vi "WPI_SolenoidSafetyCheck.vi"(0 "SolenoidDevRef":T1={"DevStatus"={"status"=FALSE, "code"=0, "source"=""}, "Pneumatics Control Module"=1, "Forward Solenoid Channel"=enum."Solenoid 1", "Reverse Solenoid Channel"=enum."Invalid"}, 5 "menu":T3, 7 "VI Refnum":refnum<vi>, 9 "timeout (ms)":u32=100, 11 "error in (no error)":errorcluster) -> (15 "error out":errorcluster)   [LabVIEW 2017]
doc: "This subVI holds an array of DevRefs, timeout values, and latest update times. These values can be added, updated, tested, and removed.\n\nThis gets called by Open to add a set of values. It gets called by Drive to update the 'last update value'. It gets called by Close to remove a set of values.\n\nIt also gets called by Safety Test via the SafetyCheckEngine that runs as a background task called by the Start Communication loop to test all sets of values for a timeout condition.\n\nThis software is licensed. Open the labview\\readme\\WPI Robotics Library Open Source License.txt file for more information."
uses:
  <vilib>/Rock Robotics/WPI/SafetyOutput/WPI_SafetyOutputCheckMenu.ctl
  <vilib>/Rock Robotics/WPI/Solenoid/WPI_SolenoidDevRef.ctl
  <vilib>/Rock Robotics/WPI/Solenoid/WPI_SolenoidChannel.ctl
  <vilib>/Rock Robotics/WPI/CAN/PCM/WPI_CAN_PCMGlobalOps.ctl
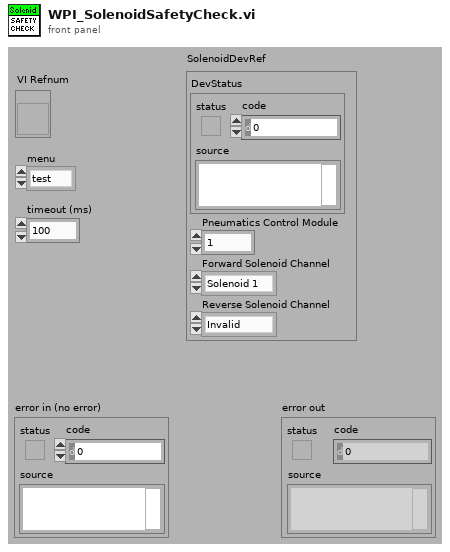
[diagram p1: front panel]
types:
  T1 = typedef "WPI_SolenoidDevRef.ctl" = cluster{"DevStatus":errorcluster, "Pneumatics Control Module":u8, "Forward Solenoid Channel":T2, "Reverse Solenoid Channel":T2}
  T2 = typedef "WPI_SolenoidChannel.ctl" = enum8{"Solenoid 0", "Solenoid 1", "Solenoid 2", "Solenoid 3", "Solenoid 4", "Solenoid 5", "Solenoid 6", "Solenoid 7", "Invalid"}
  T3 = typedef "WPI_SafetyOutputCheckMenu.ctl" = enum16{"test", "add", "remove", "update"}
  T4 = typedef "WPI_CAN_PCMGlobalOps.ctl" = enum16{"Read For Send", "Write After Receive", "Set Solenoids", "Set Closed Loop", "Clear Sticky Faults", "Get All", "Write Error", "Write After Receive Blacklist", "Set Control Frame Rate"}
  T5 = cluster{"Solenoid Status":bool[], "Battery Voltage":dbl, "Solenoid Voltage":dbl, "Compressor Current":dbl, "CompressorEnabled":bool, "StickySolenoidFault":bool, "StickyCompressorFault":bool, "SolenoidFault":bool, "CompressorFault":bool, "HardwareFault":bool, "ClosedLoopStatus":bool, "PressureStatus":bool, "Module Enabled":bool, "ClosedLoopSuggestedOutput":bool, "CAN Error":errorcluster, "Sticky Solenoid Faults":bool[]}
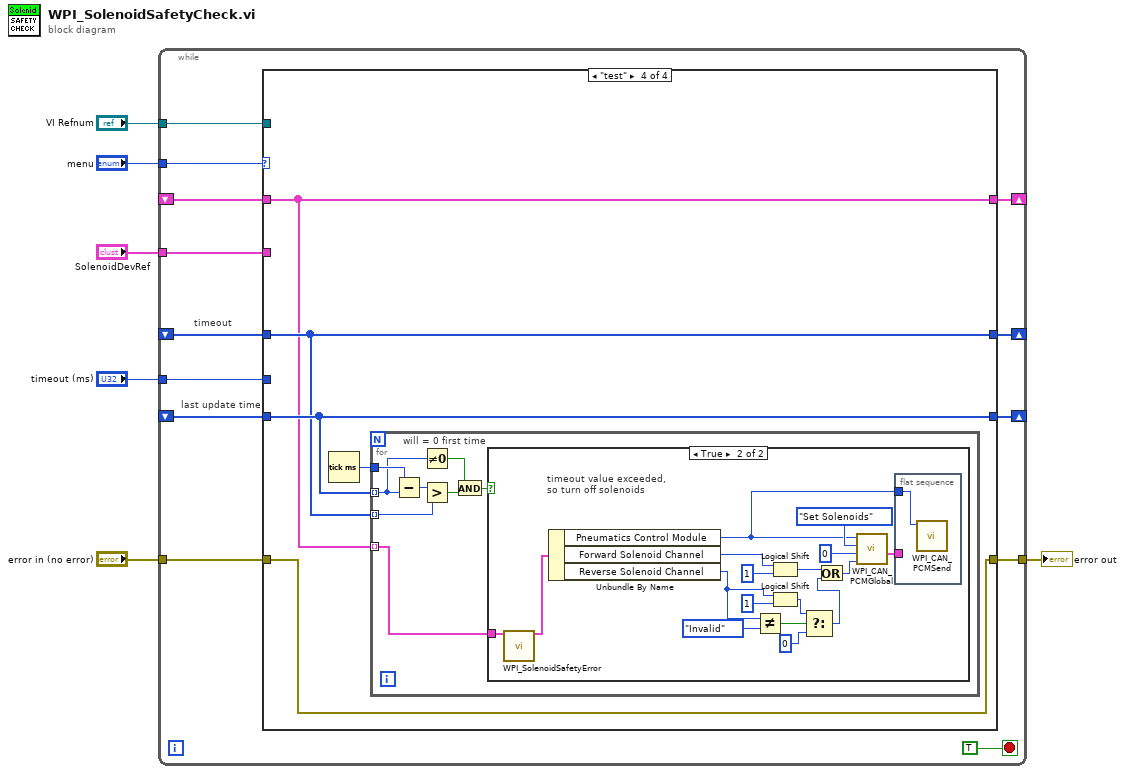
[diagram p0: block diagram]
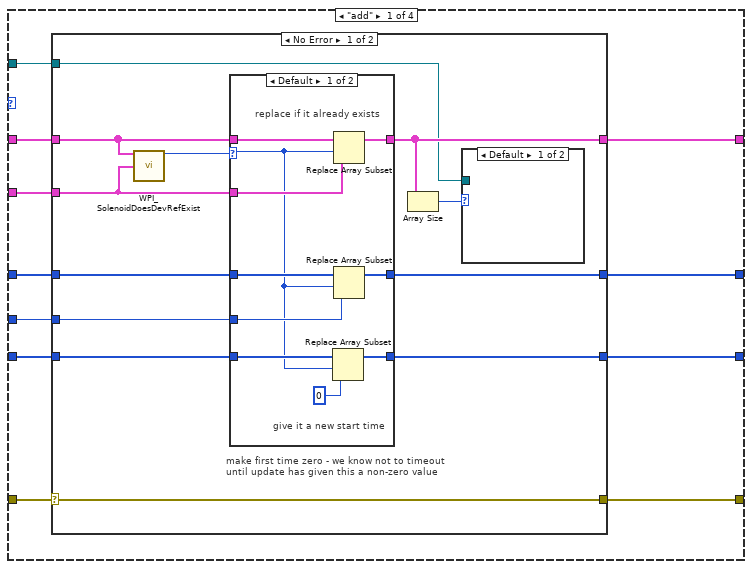
[diagram p2: hidden frame]
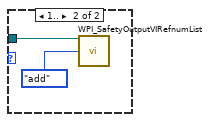
[diagram p3: hidden frame]
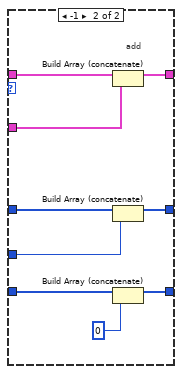
[diagram p4: hidden frame]
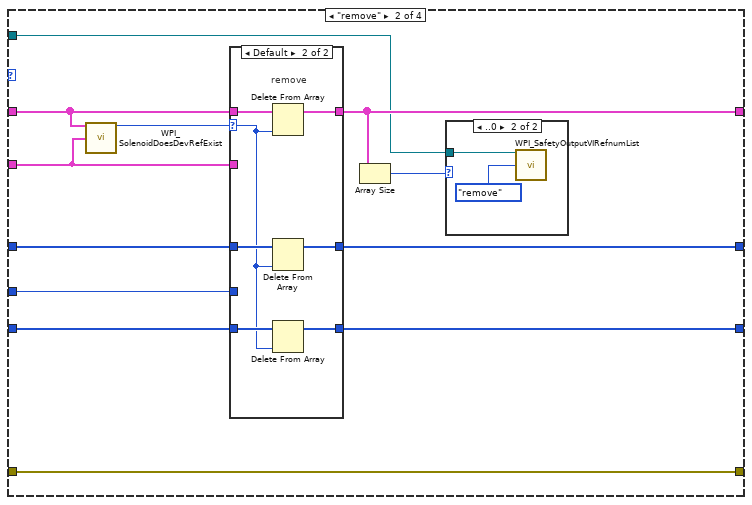
[diagram p6: hidden frame]
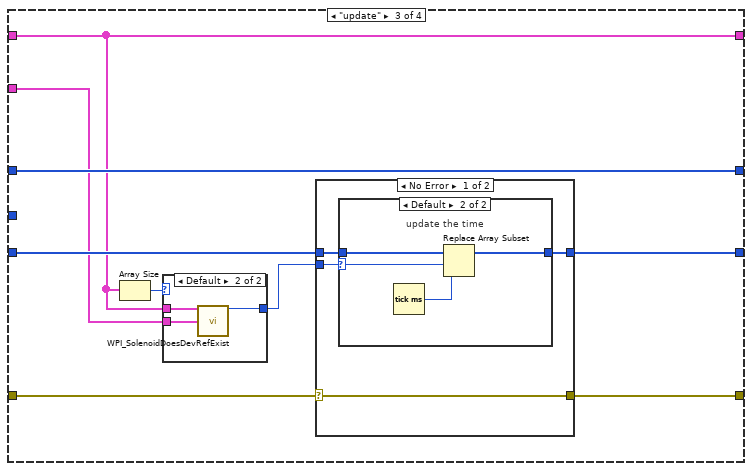
[diagram p9: hidden frame]
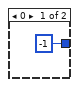
[diagram p10: hidden frame]
diagram:
  n1 = while {
    tunnel: "menu" -> [w18]
    shift-right: [w17] -> _
    shift-left: _ -> [w13]
    tunnel: "SolenoidDevRef" -> [w12]
    shift-right: [w14] -> _
    shift-left: _ -> [w16]
    tunnel: "timeout (ms)" -> [w15]
    shift-right: [w10] -> _
    shift-left: _ -> [w11]
    tunnel: "VI Refnum" -> [w9]
    tunnel: "error in (no error)" -> [w8]
    tunnel: [w7] -> w1
    stop <- TRUE stop-if-true
    # "last update time"
    # "timeout"
    n2 = case shown="\"test\"" w18 {
      tunnel: w13 -> [w30 w69 w92 w117]
      tunnel: [w23 w73 w92 w117] -> w17
      tunnel: w12 -> [w29 w68 w93 _]
      tunnel: w16 -> [w28 w79 w100 w118]
      tunnel: w15 -> [w27 w78 _ _]
      tunnel: [w26 w77 w100 w118] -> w14
      tunnel: w11 -> [w25 w76 w99 w119]
      tunnel: [w24 w75 w98 w119] -> w10
      tunnel: w9 -> [w22 w72 _ _]
      tunnel: w8 -> [w21 w71 w97 w116]
      tunnel: [w20 w71 w96 w116] -> w7
      frame "add" {
        n3 = case shown="No Error" w21 {
          selector: w21 -> [w34 w67]
          tunnel: w30 -> [w32 w66]
          tunnel: w29 -> [w31 _]
          tunnel: w28 -> [w42 w65]
          tunnel: w27 -> [w41 _]
          tunnel: [w40 w65] -> w26
          tunnel: w25 -> [w39 w64]
          tunnel: [w38 w64] -> w24
          tunnel: [w37 w66] -> w23
          tunnel: w22 -> [w36 _]
          tunnel: [w34 w67] -> w20
          frame No Error {
            # "make first time zero - we know not to timeout until update has given this a non-zero value"
            n4 = call <vilib>:"WPI_SolenoidDoesDevRefExist.vi"("SolenoidDevRefArray"=w32, "SolenoidDevRef"=w31) -> ("index"=w33:i32)  [unwired: 13 out]
            n5 = case shown="Default" w33 {
              selector: w33 -> [w46 _]
              tunnel: w32 -> [w54 w63]
              tunnel: [w53 w62] -> w37
              tunnel: w31 -> [w52 w61]
              tunnel: w42 -> [w51 w60]
              tunnel: w41 -> [w49 w59]
              tunnel: [w50 w58] -> w40
              tunnel: w39 -> [w48 w57]
              tunnel: [w47 w56] -> w38
              frame Default {
                # "give it a new start time"
                # "replace if it already exists"
                n6 = Replace Array Subset(array=w48, new element=u32 0 ("millisecond timer value"), index=w46) -> (w47:u32[])
                n7 = Replace Array Subset(array=w54, new element=w52, index=w46) -> (w53:T1[])
                n8 = Replace Array Subset(array=w51, new element=w49, index=w46) -> (w50:u32[])
              }
              frame -1 {
                # "add"
                n9 = Build Array (concatenate)(w63, w61) -> (w62:T1[])
                n10 = Build Array (concatenate)(w60, w59) -> (w58:u32[])
                n11 = Build Array (concatenate)(w57, u32 0 ("millisecond timer value")) -> (w56:u32[])
              }
            }
            n12 = Array Size(array=w37) -> (size(s)=w35:i32)
            n13 = case shown="Default" w35 {
              tunnel: w36 -> [_ w43]
              frame Default {
              }
              frame 1.. {
                n14 = call <vilib>:"WPI_SafetyOutputVIRefnumList.vi"("VI Refnum"=w43, "menu"=enum16{"read", "add", "remove"}."add") -> ()  [unwired: 14 out]
              }
            }
          }
          frame Error {
            # "do not add if there is an error"
          }
        }
      }
      frame "remove" {
        n15 = call <vilib>:"WPI_SolenoidDoesDevRefExist.vi"("SolenoidDevRefArray"=w69, "SolenoidDevRef"=w68) -> ("index"=w70:i32)  [unwired: 13 out]
        n16 = case shown="Default" w70 {
          selector: w70 -> [_ w85]
          tunnel: w69 -> [w84 w91]
          tunnel: [w84 w88] -> w73
          tunnel: w68 -> [_ _]
          tunnel: w79 -> [w83 w90]
          tunnel: w78 -> [_ _]
          tunnel: [w83 w87] -> w77
          tunnel: w76 -> [w82 w89]
          tunnel: [w82 w86] -> w75
          frame -1 {
            # "do nothing if it does not exist"
          }
          frame Default {
            # "remove"
            n17 = Delete From Array(array=w91, index=w85) -> (array with subset deleted=w88:T1[])  [unwired: 1 in, 1 out]
            n18 = Delete From Array(array=w90, index=w85) -> (array with subset deleted=w87:u32[])  [unwired: 1 in, 1 out]
            n19 = Delete From Array(array=w89, index=w85) -> (array with subset deleted=w86:u32[])  [unwired: 1 in, 1 out]
          }
        }
        n20 = Array Size(array=w73) -> (size(s)=w74:i32)
        n21 = case shown="..0" w74 {
          tunnel: w72 -> [_ w80]
          frame Default {
          }
          frame ..0 {
            n22 = call <vilib>:"WPI_SafetyOutputVIRefnumList.vi"("VI Refnum"=w80, "menu"=enum16{"read", "add", "remove"}."remove") -> ()  [unwired: 14 out]
          }
        }
      }
      frame "update" {
        n23 = Array Size(array=w92) -> (size(s)=w95:i32)
        n24 = case shown="Default" w95 {
          tunnel: [-1 ("index") w104] -> w94
          tunnel: w93 -> [_ w103]
          tunnel: w92 -> [_ w102]
          frame 0 {
          }
          frame Default {
            n25 = call <vilib>:"WPI_SolenoidDoesDevRefExist.vi"("SolenoidDevRefArray"=w102, "SolenoidDevRef"=w103) -> ("index"=w104:i32)  [unwired: 13 out]
          }
        }
        n26 = case shown="No Error" w97 {
          selector: w97 -> [w105 w115]
          tunnel: w99 -> [w108 w114]
          tunnel: [w107 w114] -> w98
          tunnel: w94 -> [w106 _]
          tunnel: [w105 w115] -> w96
          frame No Error {
            n27 = case shown="Default" w106 {
              selector: w106 -> [_ w110]
              tunnel: w108 -> [w109 w113]
              tunnel: [w109 w112] -> w107
              frame -1 {
                # "don't replace if it doesn't exist"
              }
              frame Default {
                # "update the time"
                n28 = Tick Count (ms)() -> (millisecond timer value=w111:u32)
                n29 = Replace Array Subset(array=w113, new element=w111, index=w110) -> (w112:u32[])
              }
            }
          }
          frame Error {
            # "do not update if there is an error"
          }
        }
      }
      frame "test" {
        n30 = Tick Count (ms)() -> (millisecond timer value=w120:u32)
        n31 = for {
          tunnel: w119 -> [w124] mode=indexing
          tunnel: w120 -> [w128]
          tunnel: w118 -> [w126] mode=indexing
          tunnel: w117 -> [w121] mode=indexing
          # "will = 0 first time"
          n32 = Subtract(x=w128, y=w124) -> (x-y=w127:u32)
          n33 = Not Equal To 0?(x=w124) -> (x != 0?=w122:bool)
          n34 = Greater?(x=w127, y=w126) -> (0:w125:bool)
          n35 = And(x=w122, y=w125) -> (x .and. y?=w123:bool)
          n36 = case shown="True" w123 {
            tunnel: w121 -> [_ w145]
            frame False {
              # "do nothing"
            }
            frame True {
              # "timeout value exceeded, so turn off solenoids"
              n37 = call <vilib>:"WPI_SolenoidSafetyError.vi"("SolenoidDevRef"=w145) -> ("SolenoidDevRef 2"=w142:T1)  [unwired: 14 out]
              n38 = Unbundle By Name(w142) -> ("Pneumatics Control Module"=w130:u8, "Forward Solenoid Channel"=w143:T2, "Reverse Solenoid Channel"=w137:T2)
              n39 = Not Equal?(x=w137, y=WPI_SolenoidChannel."Invalid") -> (x != y?=w135:bool)
              n40 = Logical Shift(y=w143, x=u8 1) -> (x << y=w139:u8)
              n41 = Logical Shift(y=w137, x=u8 1) -> (x << y=w134:u8)
              n42 = Select(t=w134, s=w135, f=u8 0) -> (s? t:f=w131:u8)
              n43 = Or(x=w139, y=w131) -> (x .or. y?=w132:u8)
              n44 = call <vilib>:"WPI_CAN_PCMGlobal.vi"("Solenoid Set Mask"=w132, "Solenoid Set Value"=u8 0, "Operation"=WPI_CAN_PCMGlobalOps."Set Solenoids", "Pneumatics Control Module (0)"=w130) -> ("Get All"=w129:T5)  [unwired: 5 in, 2 out]
              n45 = flat-sequence {
                tunnel: w130 -> [w146]
                tunnel: w129 -> [_]
                frame #0 {
                  n46 = call <vilib>:"WPI_CAN_PCMSend.vi"("Pneumatics Control Module (0)"=w146) -> ()  [unwired: 10 in, 1 out]
                }
              }
            }
          }
        }
      }
    }
  }
  "error out" <- w1
